vi "Buffer.New.vi"(8 "error in (no error)":errorcluster, 10 "size":u64 format="%d bytes", 11 "Buffer type":refnum<class "Buffer.lvclass">) -> (0 "error out":errorcluster, 3 "Buffer out":refnum<class "Buffer.lvclass">)   [LabVIEW 2017, in "DSF Core.lvlib" / "Buffer.lvclass"]
uses:
  Buffer.lvclass
  C:/Program Files (x86)/National Instruments/LabVIEW 2017/vi.lib/NI/Memory Manager/Classes/Pointer/Memory.Pointer.lvclass
  Buffer.lvclass/Buffer.ctl
  <vilib>/NI/Memory Manager/Classes/Pointer/Memory.Pointer.lvclass/Memory.Pointer.ctl
  <vilib>/NI/Memory Manager/Classes/Pointer/Memory.Pointer.New.1B.vi
  <vilib>/NI/Memory Manager/Classes/Pointer/Memory.Pointer.Allocate.vi
  <vilib>/NI/Memory Manager/Classes/Pointer/Memory.Pointer.Set Address.vi
  <vilib>/NI/Memory Manager/Classes/Pointer/Memory.Pointer.Set Size.vi
  <vilib>/NI/Memory Manager/Classes/Pointer/Memory.Pointer.Set Allocated.vi
  <vilib>/NI/Memory Manager/Classes/Pointer/Memory.Pointer.lvclass
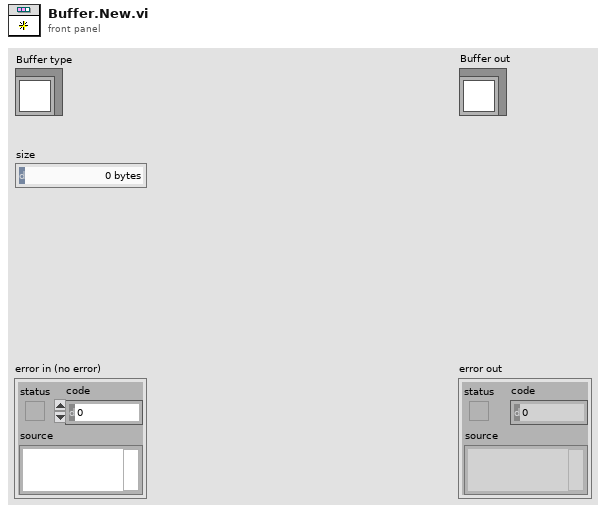
[diagram p1: front panel]
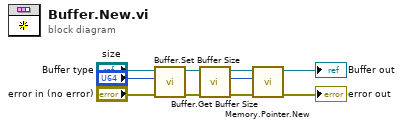
[diagram p0: block diagram]
diagram:
  n1 = call "Buffer.Set Buffer Size.vi"("buffer size"="size", "Buffer in"="Buffer type") -> ("Buffer out"=w3:refnum<class "Buffer.lvclass">)  [unwired: 9 in]
  n2 = call "Buffer.Get Buffer Size.vi"("Buffer in"=w3) -> ("buffer size"=w1:u64, "Buffer out"=w2:refnum<class "Buffer.lvclass">)  [unwired: 9 in]
  n3 = call-poly <vilib>:"Memory.Pointer.New.vi"("error in (no error)"="error in (no error)", "count (1)"=w1, "Pointer type"=w2) -> ("error out"=→"error out":errorcluster, "Pointer"=→"Buffer out":refnum<class "Buffer.lvclass">)  [unwired: 7 in]
